vi "2410C-64OutBit.vi"(8 "error in (no error)":errorcluster, 10 "BL":bool, 11 "IO_Output":T1) -> (0 "error out":errorcluster)   [LabVIEW 2015]
uses:
  Ctrl/2410C-64_SelectOutPut.ctl
  Ctrl/IO Card_Type.ctl
  global/IO_ClassTypeData.vi
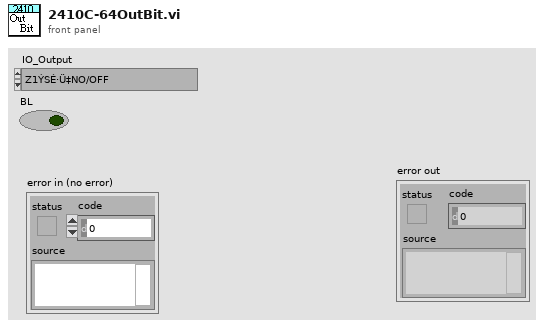
[diagram p1: front panel]
types:
  T1 = typedef "2410C-64_SelectOutPut.ctl" = enum16{"Z1ÝSÉ·Ü‡NO/OFF", "大TRAY吸取汽缸(上原位)", "´óTRAY±PÎüÈ¡Õæ¿Õ", "大TRAY破真空", "小TRAY吸取汽缸(上原位)", "Ð¡TRAY±PÎüÈ¡Õæ¿Õ", "小TRAY破真空", "ÒÆÝdÆû¸×½ÓÁÏÎ»", "ÒÆÝdÆû¸×È¡ÁÏÎ»", "大TRAY靠位汽缸", "小TRAY靠位汽缸", "收料上下汽缸(下原位)"}
  T2 = typedef "IO Card_Type.ctl" = enum16{"None", "Unidaq32", "IPC_3005(9700)", "6480", "2410C-64", "Zan"}
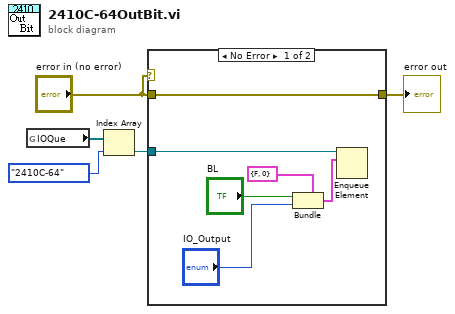
[diagram p0: block diagram]
diagram:
  n1 = global read "IO_ClassTypeData.vi" "IOQue"() -> (w3:refnum<queue>[])
  n2 = Index Array(array=w3, index=IO_Card_Type."2410C-64" ("IO Card Type")) -> (element=w1:refnum<queue>)
  n3 = case shown="No Error" "error in (no error)" {
    tunnel: "error in (no error)" -> [w6 w12]
    tunnel: [w6 w12] -> w5
    tunnel: w1 -> [w11 _]
    frame No Error {
      n4 = Bundle(cluster=cluster{"BL":bool, "Index":i32} {"BL"=FALSE, "Index"=0} ("element"), "BL"="BL", "Index"="IO_Output") -> (w8:cluster{"BL":bool, "Index":i32})
      n5 = Enqueue Element(queue=w11, element=w8) -> ()  [unwired: 2 in, 3 out]
    }
    frame Error {
    }
  }
  "error out" <- w5
